vi "SeCrTs-Irms_Module_L.vi"(7 "Data FIFO Ref":T1, 8 "error in":errorcluster, 11 "TCP Network Connection in":refnum<k5>) -> (0 "error out":errorcluster, 3 "TCP Network Connection out":refnum<k5>)   [LabVIEW 2022 SP3]
uses:
  RT Controls/SeCrTs-Data FIFO.ctl
  <vilib>/Analysis/3filter.llb/Filter Passband Type.ctl
  <vilib>/Analysis/NI_AALBase.lvlib
  <vilib>/ptbypt/NI_PtbyPt.lvlib
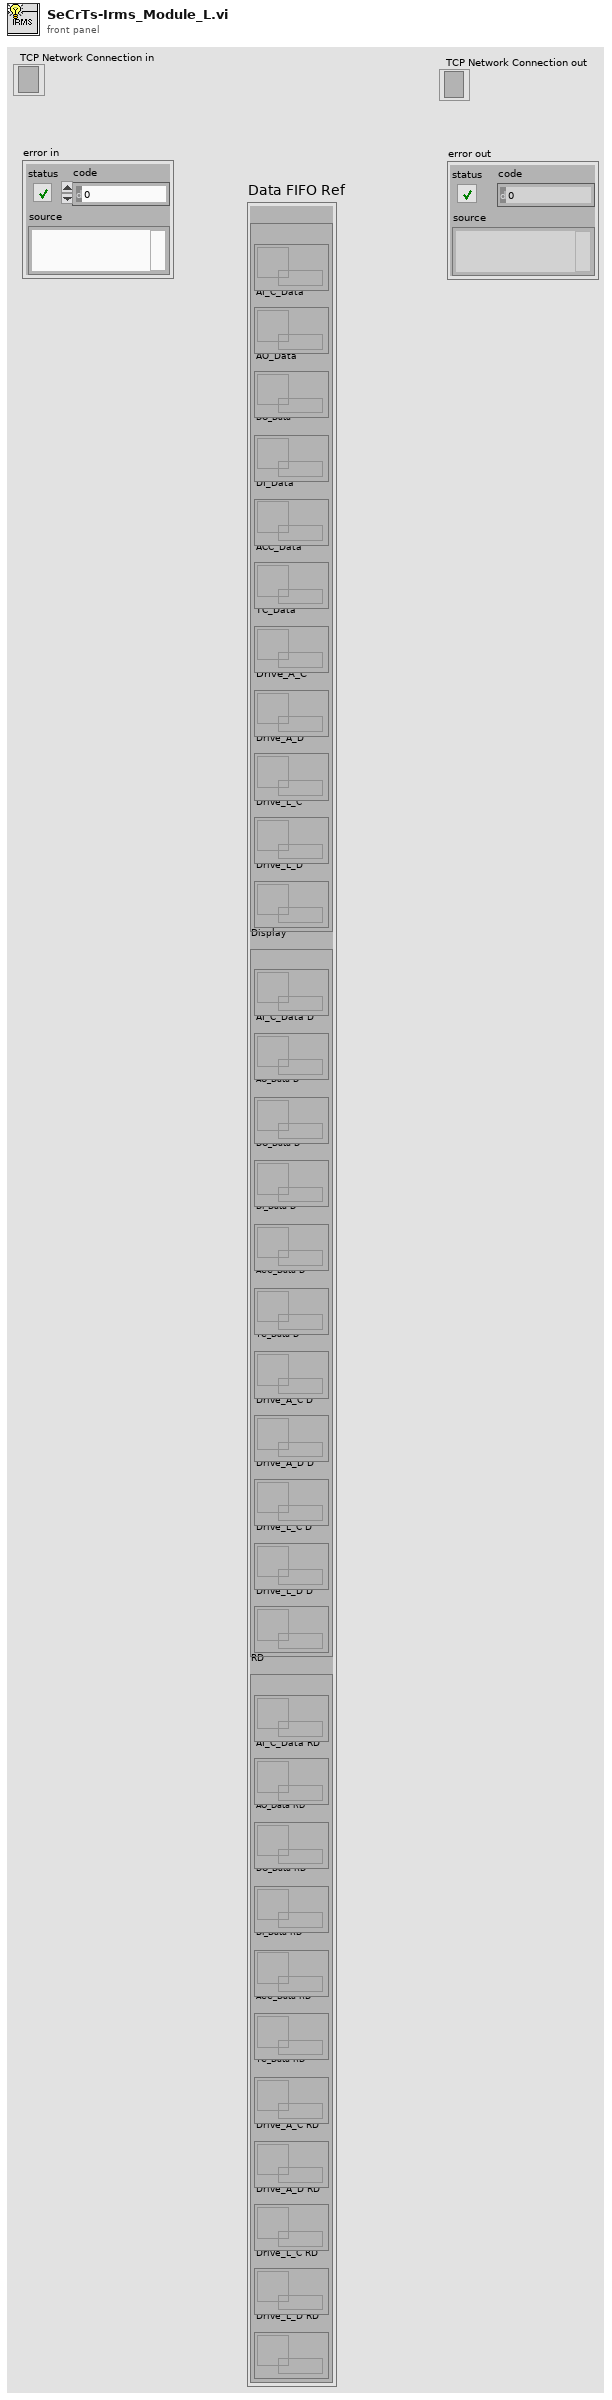
[diagram p1: front panel]
types:
  T1 = typedef "SeCrTs-Data FIFO.ctl" = cluster{"Control":cluster{"AI_V_Data":refnum<queue>, "AI_C_Data":refnum<queue>, "AO_Data":refnum<queue>, "DO_Data":refnum<queue>, "DI_Data":refnum<queue>, "ACC_Data":refnum<queue>, "TC_Data":refnum<queue>, "Drive_A_C":refnum<queue>, "Drive_A_D":refnum<queue>, "Drive_L_C":refnum<queue>, "Drive_L_D":refnum<queue>}, "Display":cluster{"AI_V_Data D":refnum<queue>, "AI_C_Data D":refnum<queue>, "AO_Data D":refnum<queue>, "DO_Data D":refnum<queue>, "DI_Data D":refnum<queue>, "ACC_Data D":refnum<queue>, "TC_Data D":refnum<queue>, "Drive_A_C D":refnum<queue>, "Drive_A_D D":refnum<queue>, "Drive_L_C D":refnum<queue>, "Drive_L_D D":refnum<queue>}, "RD":cluster{"AI_V_Data RD":refnum<queue>, "AI_C_Data RD":refnum<queue>, "AO_Data RD":refnum<queue>, "DO_Data RD":refnum<queue>, "DI_Data RD":refnum<queue>, "ACC_Data RD":refnum<queue>, "TC_Data RD":refnum<queue>, "Drive_A_C RD":refnum<queue>, "Drive_A_D RD":refnum<queue>, "Drive_L_C RD":refnum<queue>, "Drive_L_D RD":refnum<queue>}}
  T2 = typedef "NI_AALBase.lvlib/Filter Passband Type.ctl" = enum32{"Lowpass", "Highpass", "Bandpass", "Bandstop"}
  T3 = cluster{"En_Drive_A":bool, "En_Drive_L":bool, "Exit_Drive_A":bool, "Exit_Drive_L":bool}
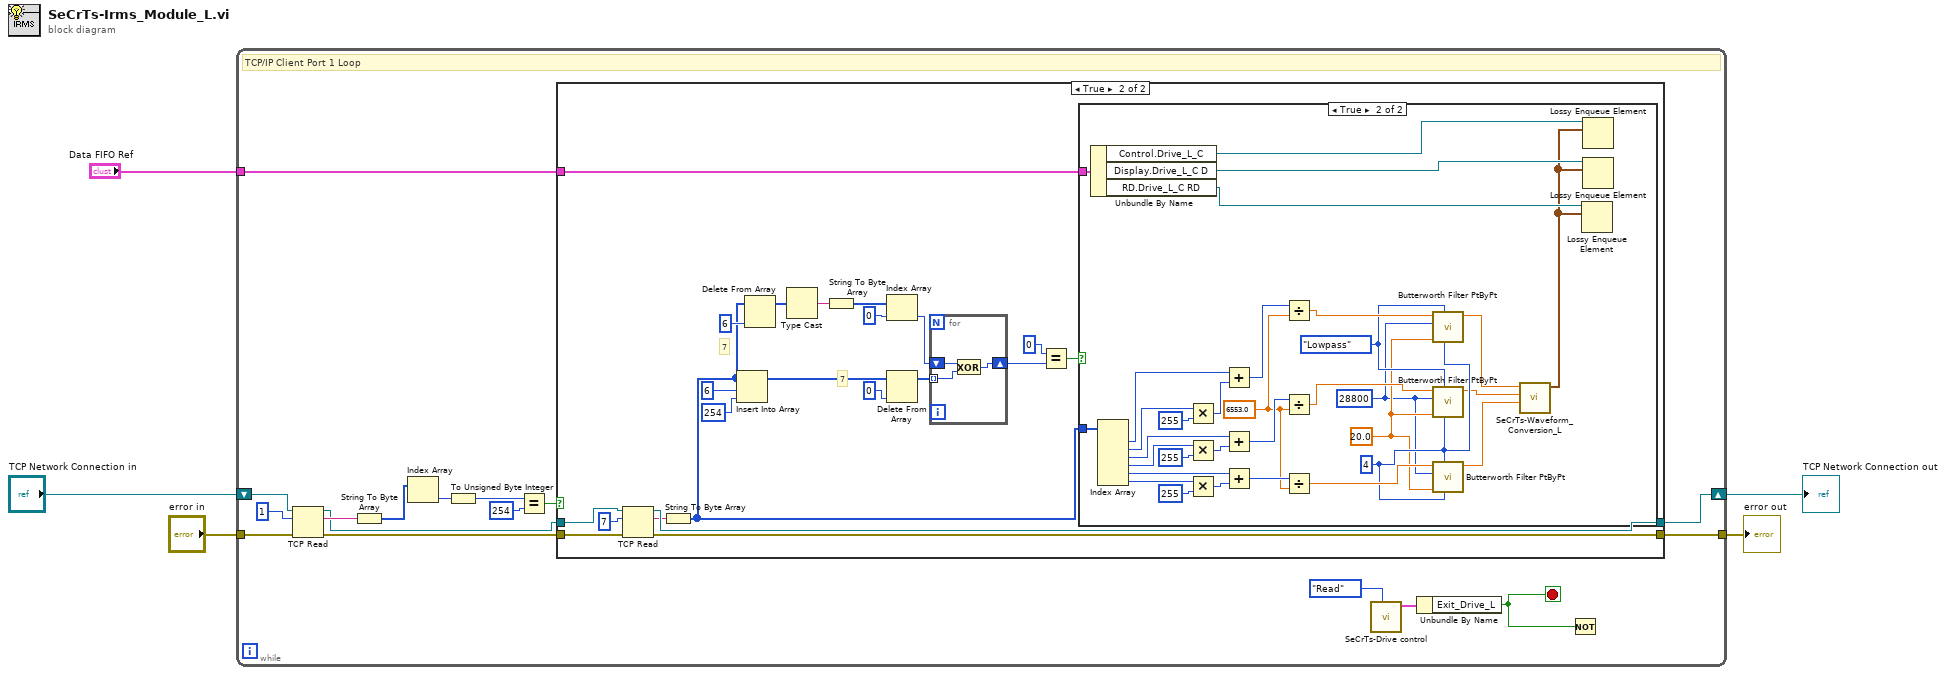
[diagram p0: block diagram]
diagram:
  n1 = while {
    tunnel: [w14] -> w3
    shift-right: [w13] -> w4
    shift-left: "TCP Network Connection in" -> [w22]
    tunnel: "error in" -> [w10]
    tunnel: "Data FIFO Ref" -> [w9]
    stop <- w6 stop-if-true
    # "TCP/IP Client Port 1 Loop"
    n2 = TCP Read(connection ID=w22, bytes to read=1, error in (no error)=w10) -> (connection ID out=w15:refnum<k5>, data out=w16:string, error out=w11:errorcluster)  [unwired: 2 in]
    n3 = String To Byte Array(string=w16) -> (unsigned byte array=w20:u8[])
    n4 = Index Array(array=w20) -> (element=w19:u8)  [unwired: 1 in]
    n5 = To Unsigned Byte Integer(number=w19) -> (unsigned 8bit integer=w18:u8)
    n6 = Equal?(x=w18, y=u8 254) -> (x = y?=w12:bool)
    n7 = case shown="True" w12 {
      tunnel: w15 -> [w23 w46]
      tunnel: w11 -> [w24 w45]
      tunnel: [w24 w44] -> w14
      tunnel: [w23 w43] -> w13
      tunnel: w9 -> [_ w25]
      frame False {
      }
      frame True {
        # "7"
        # "7"
        n8 = TCP Read(connection ID=w46, bytes to read=7, error in (no error)=w45) -> (connection ID out=w43:refnum<k5>, data out=w42:string, error out=w44:errorcluster)  [unwired: 2 in]
        n9 = String To Byte Array(string=w42) -> (unsigned byte array=w29:u8[])
        n10 = Insert Into Array(array=w29, index=6, new element=u8 254 ("new element/subarray")) -> (w30:u8[])
        n11 = Delete From Array(array=w29, index=6) -> (array with subset deleted=w33:u8[])  [unwired: 1 in, 1 out]
        n12 = Type Cast(x=w33) -> (*(type *) &x=w39:string)  [unwired: 1 in]
        n13 = String To Byte Array(string=w39) -> (unsigned byte array=w34:u8[])
        n14 = Index Array(array=w34, index=0) -> (element=w37:u8)
        n15 = Delete From Array(array=w30, index=0) -> (array with subset deleted=w36:u8[])  [unwired: 1 in, 1 out]
        n16 = for {
          shift-right: [w80] -> w27
          shift-left: w37 -> [w81]
          tunnel: w36 -> [w79] mode=indexing
          n17 = Exclusive Or(1:w79, 2:w81) -> (0:w80:u8)
        }
        n18 = Equal?(x=u8 0, y=w27) -> (x = y?=w26:bool)
        n19 = case shown="True" w26 {
          tunnel: w29 -> [_ w63]
          tunnel: w25 -> [_ w51]
          frame False {
          }
          frame True {
            w58 = Filter_Passband_Type."Lowpass" ("filter type")
            w57 = 4 ("order")
            w56 = 20.0 ("low cutoff freq: fl")
            w55 = 28800 ("rank")
            w62 = 6553.0
            n20 = Unbundle By Name(w51) -> ("Control.Drive_L_C"=w50:refnum<queue>, "Display.Drive_L_C D"=w49:refnum<queue>, "RD.Drive_L_C RD"=w48:refnum<queue>)
            n21 = Index Array(array=w63) -> (element #1=w76:u8, element #2=w75:u8, element #3=w70:u8, element #4=w69:u8, element #5=w68:u8, element #6=w67:u8)  [unwired: 6 in]
            n22 = Multiply(x=w75, y=u32 255) -> (x*y=w77:u32)
            n23 = Multiply(x=w69, y=u32 255) -> (x*y=w74:u32)
            n24 = Multiply(x=w67, y=u32 255) -> (x*y=w71:u32)
            n25 = Add(x=w76, y=w77) -> (x+y=w66:u32)
            n26 = Add(x=w70, y=w74) -> (x+y=w65:u32)
            n27 = Add(x=w68, y=w71) -> (x+y=w64:u32)
            n28 = Divide(x=w66, y=w62) -> (x/y=w61:dbl)
            n29 = Divide(x=w65, y=w62) -> (x/y=w60:dbl)
            n30 = Divide(x=w64, y=w62) -> (x/y=w59:dbl)
            n31 = call <vilib>:"Butterworth Filter PtByPt.vi"("order"=w57, "filter type"=w58, "low cutoff freq: fl"=w56, "sampling freq: fs"=w55, "x"=w61) -> ("Filtered x"=w54:dbl)  [unwired: 4 in, 1 out]
            n32 = call <vilib>:"Butterworth Filter PtByPt.vi"("order"=w57, "filter type"=w58, "low cutoff freq: fl"=w56, "sampling freq: fs"=w55, "x"=w60) -> ("Filtered x"=w53:dbl)  [unwired: 4 in, 1 out]
            n33 = call <vilib>:"Butterworth Filter PtByPt.vi"("order"=w57, "filter type"=w58, "low cutoff freq: fl"=w56, "sampling freq: fs"=w55, "x"=w59) -> ("Filtered x"=w52:dbl)  [unwired: 4 in, 1 out]
            n34 = call "SeCrTs-Waveform_Conversion_L.vi"("Irms3"=w52, "Irms2"=w53, "Irms1"=w54) -> ("Array"=w47:waveform(dbl)[])  [unwired: 8 in]
            n35 = Lossy Enqueue Element(queue=w48, element=w47) -> ()  [unwired: 1 in, 4 out]
            n36 = Lossy Enqueue Element(queue=w50, element=w47) -> ()  [unwired: 1 in, 4 out]
            n37 = Lossy Enqueue Element(queue=w49, element=w47) -> ()  [unwired: 1 in, 4 out]
          }
        }
      }
    }
    n38 = call "SeCrTs-Drive control.vi"("Action"=enum16{"Init", "Write", "Read"}."Read") -> ("Loop Control Out"=w7:T3)  [unwired: 9 in, 1 out]
    n39 = Unbundle By Name(w7) -> ("Exit_Drive_L"=w6:bool)
    n40 = Not(x=w6) -> ()  [unwired: 1 out]
  }
  "TCP Network Connection out" <- w4
  "error out" <- w3
